vi "FPS Monitor.vi"() -> ()   [LabVIEW 2017]
panel:
  out "FPS":dbl
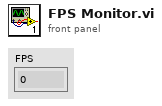
[diagram p1: front panel]
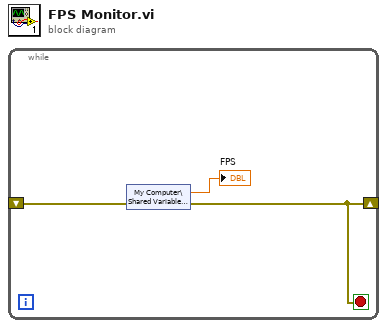
[diagram p0: block diagram]
diagram:
  n1 = while {
    shift-right: [w1] -> _
    shift-left: _ -> [w2]
    stop <- w1 stop-if-true
    n2 = shared-variable "My Computer\\Shared Variables Library.lvlib\\FPS"(error in=w2) -> (→"FPS":dbl, error out=w1:errorcluster)
  }
